vi "Draw.vi"(7 "menu in":refnum<class "menu.lvclass">, 8 "error in (no error)":errorcluster, 11 "menu item in":refnum<class "menu item.lvclass">) -> (0 "error out":errorcluster, 3 "menu item out":refnum<class "menu item.lvclass">)   [LabVIEW 2009, in "menu item.lvclass"]
uses:
  menu item.lvclass
  Menu/menu.lvclass
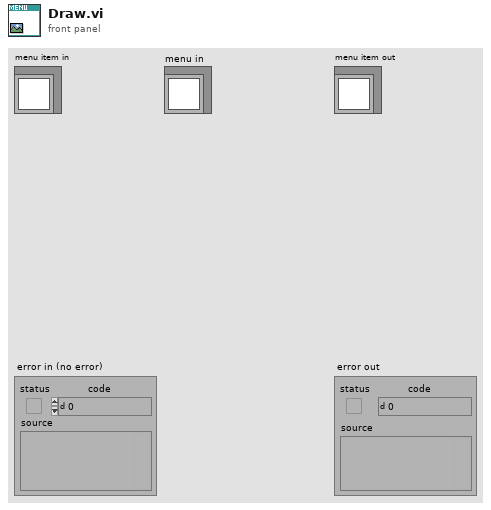
[diagram p1: front panel]
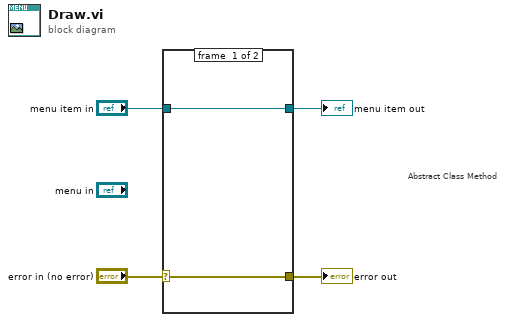
[diagram p0: block diagram]
diagram:
  # "Abstract Class Method"
  n1 = case shown="No Error" "error in (no error)" {
    selector: "error in (no error)" -> [w5 w8]
    tunnel: [w5 w8] -> w2
    tunnel: [w6 w7] -> w4
    tunnel: "menu item in" -> [w6 w7]
    frame #0 {
    }
    frame #1 {
    }
  }
  "menu item out" <- w4
  "error out" <- w2
